vi "备选颜色.vi"(10 "索引2":enum16{"空白", "蛇", "食物", "墙", "传送门"}(ring), 11 "颜色1":u32(colorbox)) -> (2 "颜色2":u32(colorbox), 3 "索引1":enum16{"空白", "蛇", "食物", "墙", "传送门"}(ring))   [LabVIEW 2012]
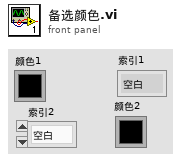
[diagram p1: front panel]
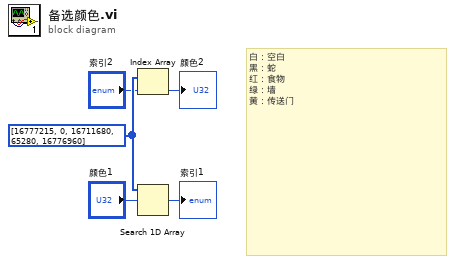
[diagram p0: block diagram]
diagram:
  w3 = u32[] [16777215, 0, 16711680, 65280, 16776960]
  # "白：空白\n黑：蛇\n红：食物\n绿：墙\n黄：传送门"
  n1 = Index Array(array=w3, index="索引2") -> (element=→"颜色2":u32)
  n2 = Search 1D Array(1D array=w3, element="颜色1") -> (index of element=→"索引1":i32)  [unwired: 1 in]
